vi "ExampleBasic64.vi"() -> ()   [LabVIEW 2009]
panel:
  in  "Device":i32 min=1 max=2
  in  "Set Device":bool
  out "Initializing":bool
  in  "STOP if TRUE":bool
  out "Focal tilt":dbl format="%.2f"
  out "Angular deviation":dbl format="%.2f"
  out "Focal length":dbl format="%.2f"
  out "Serial Number":string
  out "No of devices":i32
  out "GetOpticalParameters":string
  out "GetSerialNumber":string
  out "GetNumberDevices":string
  out "Close":string
  out "Initialize":string
  # "INITIALIZATION"
  # "SDK RETURN VALUES"
  # "SHAMROCK PARAMETERS"
  # "ACTIONS"
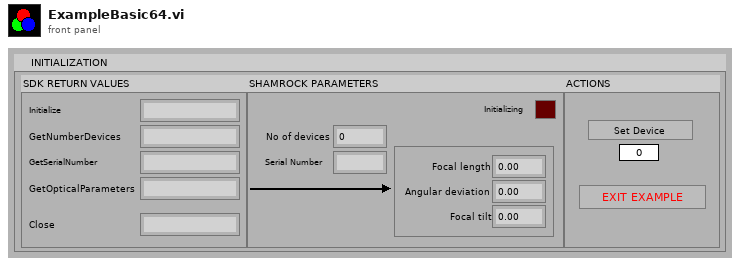
[diagram p1: front panel]
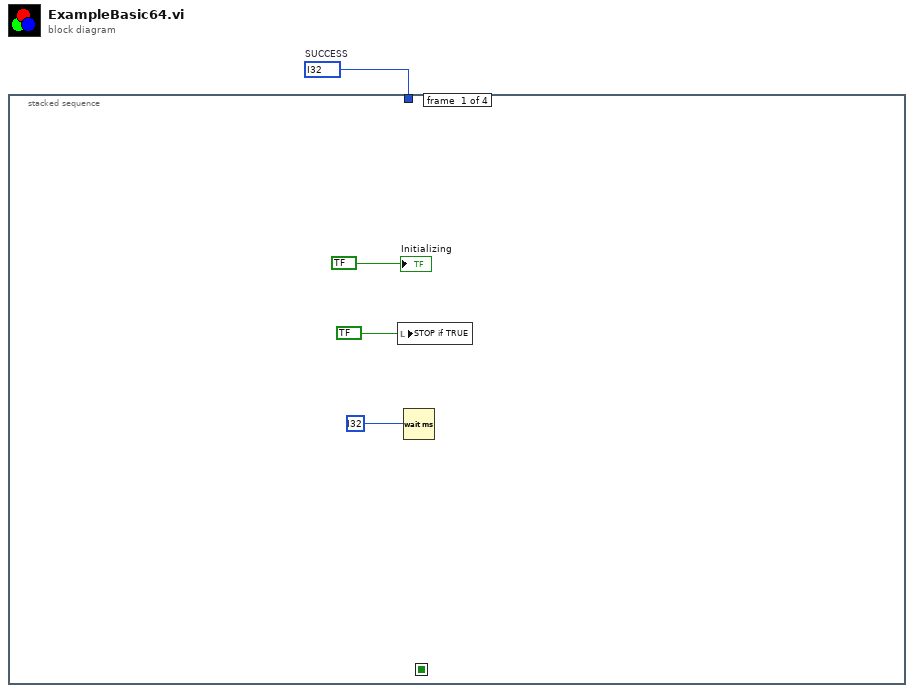
[diagram p0: block diagram]
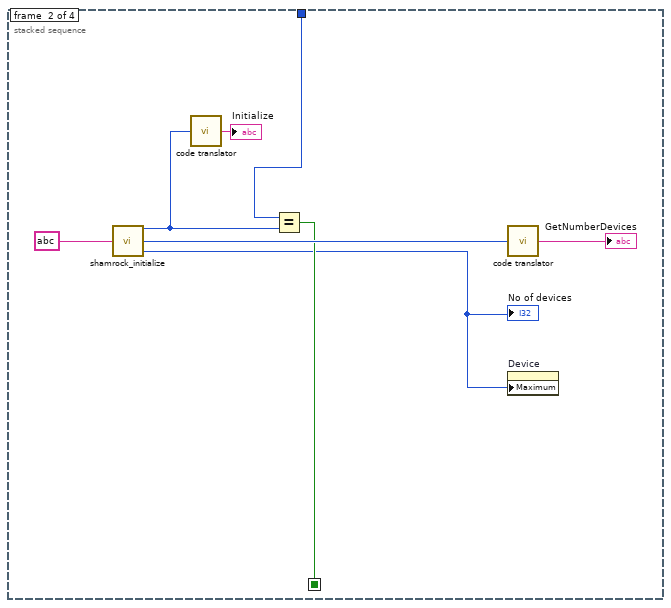
[diagram p2: hidden frame]
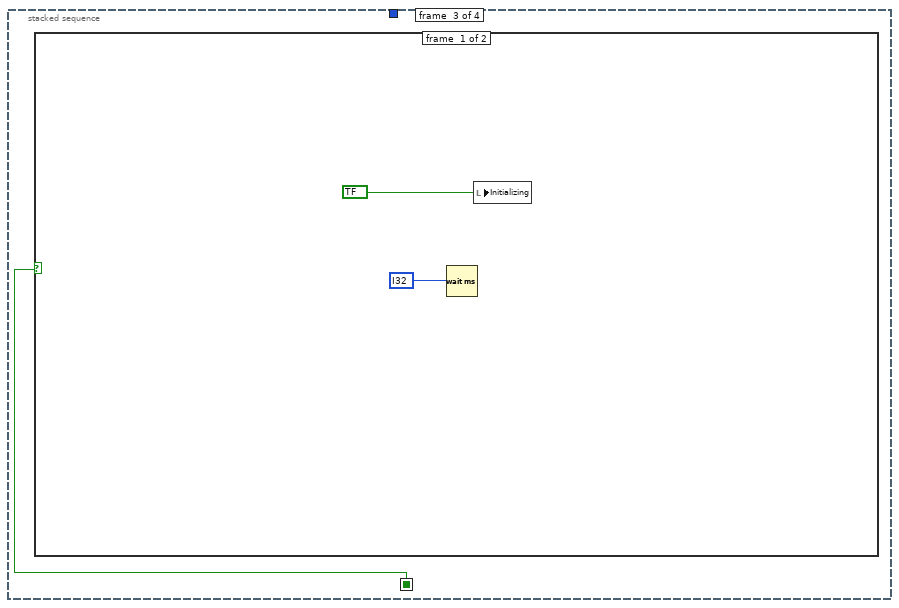
[diagram p3: hidden frame]
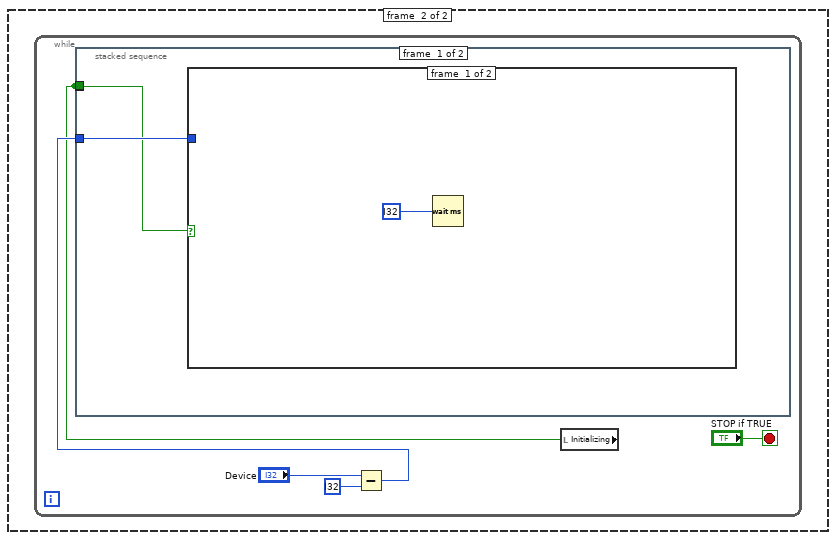
[diagram p4: hidden frame]
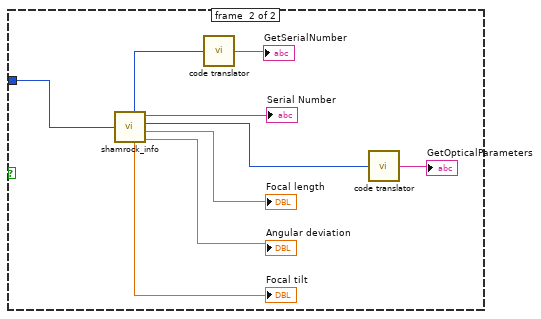
[diagram p5: hidden frame]
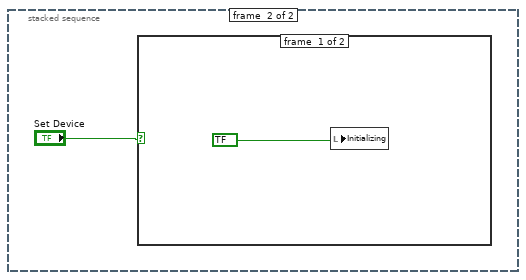
[diagram p6: hidden frame]
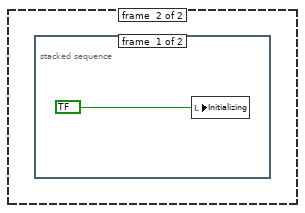
[diagram p7: hidden frame]
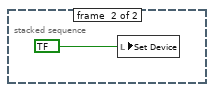
[diagram p8: hidden frame]
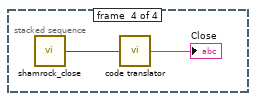
[diagram p9: hidden frame]
diagram:
  w1 = i32 ?  # SUCCESS
  n1 = stacked-sequence {
    seq-local: [_ w6 _ _] -> [_ _ w13 _]
    tunnel: w1 -> [_ w12 _ _]
    frame #0 {
      n2 = local write "STOP if TRUE"(bool ?) -> ()
      n3 = Wait (ms)(milliseconds to wait=i32 ?) -> ()  [unwired: 1 out]
      "Initializing" <- bool ?
    }
    frame #1 {
      n4 = call <userlib>:"shamrock_initialize.vi"("Initialization path"=string ?) -> ("Initialize"=w9:u32, "GetNumberDevices"=w8:u32, "No of devices"=w5:i32)
      "No of devices" <- w5
      n5 = call <userlib>:"code translator.vi"("Error code"=w9) -> ("Error description"=→"Initialize":string)
      n6 = Equal?(x=w12, y=w9) -> (x = y?=w6:bool)
      n7 = call <userlib>:"code translator.vi"("Error code"=w8) -> ("Error description"=→"GetNumberDevices":string)
      n8 = property on="Device" class="DigNum (strict)"("Maximum"=w5) -> ()  [unwired: 2 in, 2 out]
    }
    frame #2 {
      n9 = case shown="True" w13 {
        frame #0 {
          n10 = Wait (ms)(milliseconds to wait=i32 ?) -> ()  [unwired: 1 out]
          n11 = local write "Initializing"(bool ?) -> ()
        }
        frame #1 {
          n12 = while {
            stop <- "STOP if TRUE" stop-if-true
            n13 = Subtract(x="Device", y=i32 ?) -> (x-y=w19:i32)
            n14 = local read "Initializing"() -> (w16:bool)
            n15 = stacked-sequence {
              tunnel: w19 -> [w22 _]
              tunnel: w16 -> [w21 _]
              tunnel: w16 -> [_ _]
              frame #0 {
                n16 = case shown="True" w21 {
                  tunnel: w22 -> [_ w24]
                  frame #0 {
                    n17 = Wait (ms)(milliseconds to wait=i32 ?) -> ()  [unwired: 1 out]
                  }
                  frame #1 {
                    n18 = call <userlib>:"shamrock_info.vi"("Device No"=w24) -> ("GetSerialNumber"=w28:u32, "Focal tilt"=→"Focal tilt":sgl, "Serial Number"=→"Serial Number":string, "GetOpticalParameters"=w26:u32, "Focal length"=→"Focal length":sgl, "Angular deviation"=→"Angular deviation":sgl)
                    n19 = call <userlib>:"code translator.vi"("Error code"=w28) -> ("Error description"=→"GetSerialNumber":string)
                    n20 = call <userlib>:"code translator.vi"("Error code"=w26) -> ("Error description"=→"GetOpticalParameters":string)
                  }
                }
              }
              frame #1 {
                n21 = case shown="True" "Set Device" {
                  frame #0 {
                    n22 = local write "Initializing"(bool ?) -> ()
                  }
                  frame #1 {
                    n23 = stacked-sequence {
                      frame #0 {
                        n24 = local write "Initializing"(bool ?) -> ()
                      }
                      frame #1 {
                        n25 = local write "Set Device"(bool ?) -> ()
                      }
                    }
                  }
                }
              }
            }
          }
        }
      }
    }
    frame #3 {
      n26 = call <userlib>:"shamrock_close.vi"() -> ("Close"=w38:u32)
      n27 = call <userlib>:"code translator.vi"("Error code"=w38) -> ("Error description"=→"Close":string)
    }
  }
